vi "Loop Timer.vi"(1 "Wait time":u32=30) -> (0 "Loop Time":u32=31)   [LabVIEW 2018]
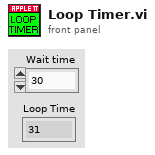
[diagram p1: front panel]
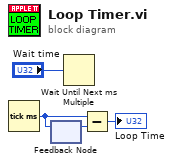
[diagram p0: block diagram]
diagram:
  n1 = Tick Count (ms)() -> (millisecond timer value=w2:u32)
  n2 = feedback #1() -> (w3:u32)  [unwired: 1 in]
  n3 = feedback-in #1(w2) -> ()
  n4 = Wait Until Next ms Multiple(millisecond multiple="Wait time") -> ()  [unwired: 1 out]
  n5 = Subtract(x=w2, y=w3) -> (x-y=→"Loop Time":u32)
